vi "ResetPack.vi"(0 "handle in":i32, 1 "UnitAddress(0)":u16, 5 "error in":errorcluster) -> (14 "handle out":i32, 19 "error out":errorcluster)   [LabVIEW 2014, in "Sixpack - Driver.lvlib"]
doc: "ACHTUNG: Alle eingestellten Parameter gehen verloren und werden durch Defaultwerte ersetzt! Dieses Kommando dauert ungefähr 1 Sekunde.\n\nAnmerkung: Über RS232 wird währenddessen ein 0-Byte empfangen."
uses:
  Sixpack - Driver.lvlib
  DLL/PackDLL.dll
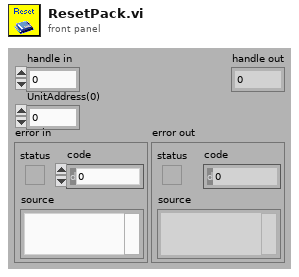
[diagram p1: front panel]
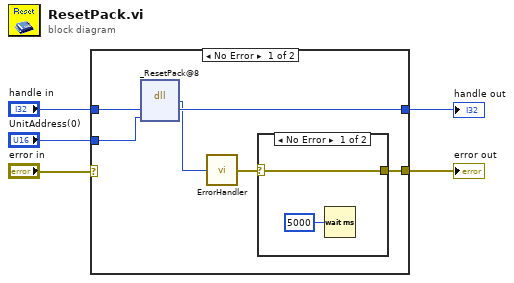
[diagram p0: block diagram]
diagram:
  n1 = case shown="No Error" "error in" {
    selector: "error in" -> [_ w16]
    tunnel: "handle in" -> [w11 w15]
    tunnel: [w10 w15] -> w4
    tunnel: "UnitAddress(0)" -> [w9 _]
    tunnel: [w6 w16] -> w2
    frame No Error {
      n2 = dll-call lib="D:/CS-Source/LV2014/GPL/instr.lib/SixPack/PackDLL/DLL/PackDLL.dll" fn="_ResetPack@8" label="ResetPack"("HANDLE"=w11, "UnitAddress"=w9) -> ("BOOLEAN"=w8:i8, "HANDLE"=w10:i32)  [unwired: 4 in, 2 out]
      n3 = call "ErrorHandler.vi"("BOOLEAN"=w8) -> ("error out"=w7:errorcluster)
      n4 = case shown="No Error" w7 {
        selector: w7 -> [w12 w14]
        tunnel: [w12 w14] -> w6
        frame No Error {
          n5 = Wait (ms)(milliseconds to wait=u32 5000) -> ()  [unwired: 1 out]
        }
        frame Error {
        }
      }
    }
    frame Error {
    }
  }
  "handle out" <- w4
  "error out" <- w2
